vi "Close.vi"(8 "error in (no error)":errorcluster, 11 "HAMAMATSU_DCAMAPI in":refnum<class "HAMAMATSU_DCAMAPI.lvclass">) -> (0 "error out":errorcluster, 3 "HAMAMATSU_DCAMAPI out":refnum<class "HAMAMATSU_DCAMAPI.lvclass">)   [LabVIEW 2020, in "HAMAMATSU_DCAMAPI.lvclass"]
uses:
  HAMAMATSU_DCAMAPI.lvclass
  HAMAMATSU_DCAMAPI.lvclass/HAMAMATSU_DCAMAPI.ctl
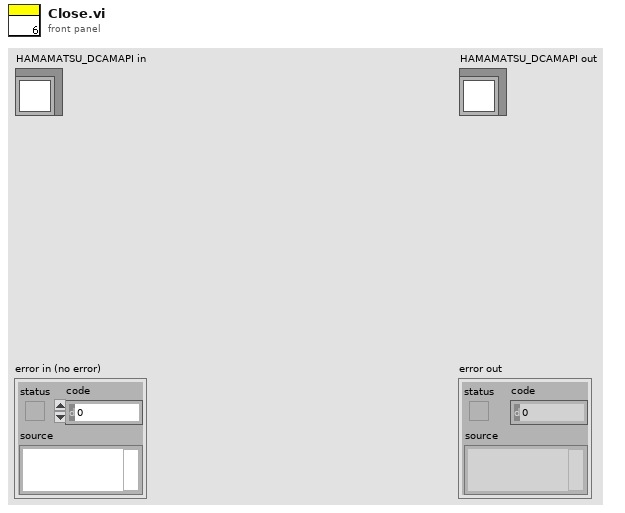
[diagram p1: front panel]
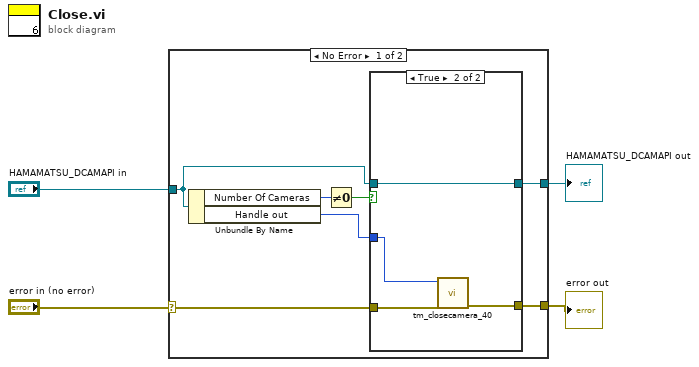
[diagram p0: block diagram]
diagram:
  n1 = case shown="No Error" "error in (no error)" {
    selector: "error in (no error)" -> [w11 w19]
    tunnel: "HAMAMATSU_DCAMAPI in" -> [w8 w18]
    tunnel: [w10 w19] -> w2
    tunnel: [w9 w18] -> w1
    frame No Error {
      n2 = Unbundle By Name(w8) -> ("Number Of Cameras"=w7:u32, "Handle out"=w5:u32)
      n3 = Not Equal To 0?(x=w7) -> (x != 0?=w6:bool)
      n4 = case shown="True" w6 {
        tunnel: w11 -> [w12 w16]
        tunnel: [w12 w15] -> w10
        tunnel: w8 -> [w13 w17]
        tunnel: [w13 w17] -> w9
        tunnel: w5 -> [_ w14]
        frame False {
        }
        frame True {
          n5 = call <userlib>:"tm_closecamera_40.vi"("error in (no error)"=w16, "Handle in"=w14) -> ("error out"=w15:errorcluster)  [unwired: 9 in]
        }
      }
    }
    frame Error {
    }
  }
  "error out" <- w2
  "HAMAMATSU_DCAMAPI out" <- w1
